vi "Set_Tunnel_Speed_server.vi"(3 "Tunnel Velocity m/s":dbl min=0.0 max=50.0 format="%.2f", 4 "Rig Name":string, 5 "Mode":T1, 6 "Client Name":string="G3_3 HD") -> (0 "Error String":string, 1 "Settling Time (s)":dbl format="%.2f", 2 "Valid Client":bool)   [LabVIEW 2013]
uses:
  ADAM Client/Sub VIs/ADAM Controls/Tunnel_speed_mode.ctl
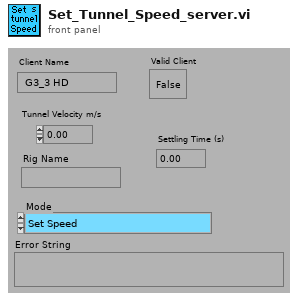
[diagram p1: front panel]
types:
  T1 = typedef "Tunnel_speed_mode.ctl" = enum16{"Set Speed", "Set Speed then wait", "Is tunnel speed allowable?"}
  T2 = typedef "Ch_description_ADAM.ctl" = cluster{"Ch Name":string, "Type":T3, "Function":T4, "Ch State":T5, "Calibration type":T6, "A":dbl, "B":dbl, "C":dbl, "D":dbl, "Comments":string, "Address":T7, "String":string, "Duty":u16}
  T3 = typedef "Module_type_ADAM.ctl" = string
  T4 = typedef "Function_ADAM.ctl" = enum16{"Analogue Input", "Digital Input", "Event counter", "Event rate", "Analogue Output", "Digital Output", "Relay Output"}
  T5 = typedef "Channel_State.ctl" = enum16{"On", "Off", "Always On", "Always Off"}
  T6 = typedef "Calib_type_ADAM.ctl" = enum16{"Raw", "Bx + A", "Cx^2 + Bx + A", "Dx^3 + Cx^2 + Bx + A", "In Band", "Hi-Tec Q", "Hi-Tec M_dot", "Text"}
  T7 = typedef "Address.ctl" = cluster{"Main":i32, "Ch.":i32, "Sub":i32, "Port Name":string}
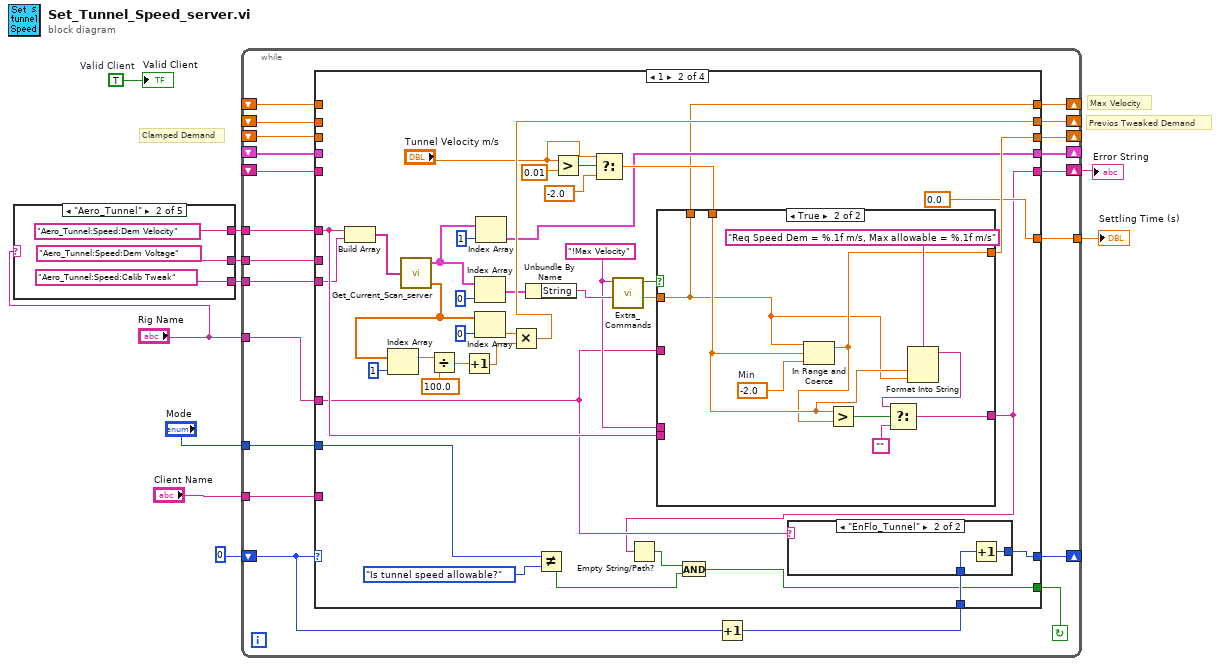
[diagram p0: block diagram]
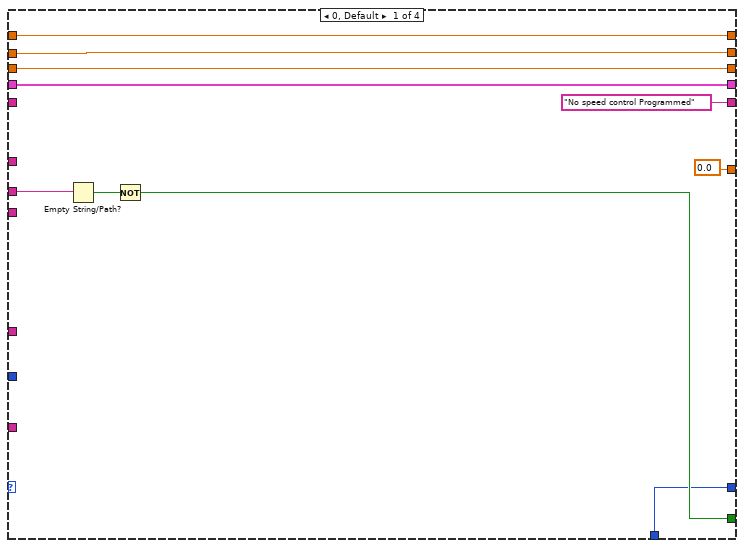
[diagram p2: hidden frame]
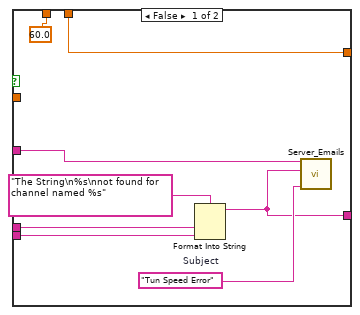
[diagram p4: hidden frame]
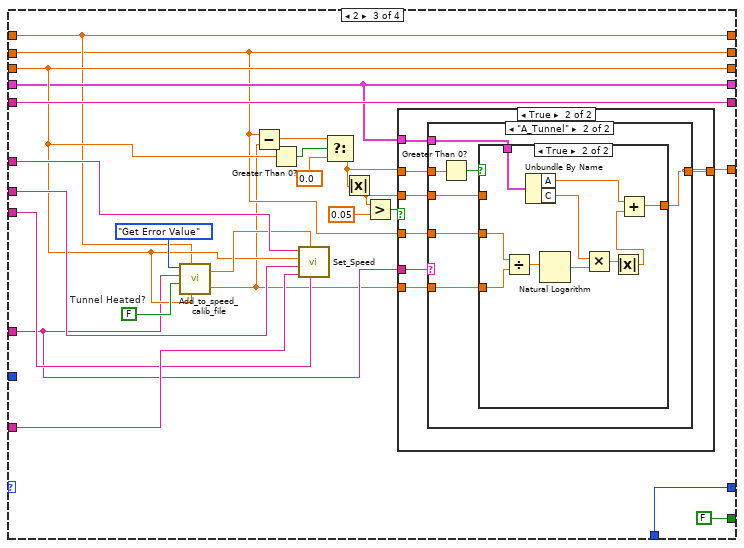
[diagram p5: hidden frame]
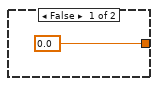
[diagram p6: hidden frame]
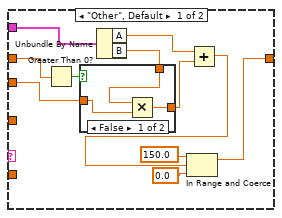
[diagram p7: hidden frame]
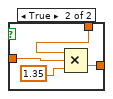
[diagram p8: hidden frame]
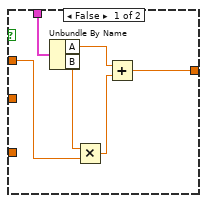
[diagram p9: hidden frame]
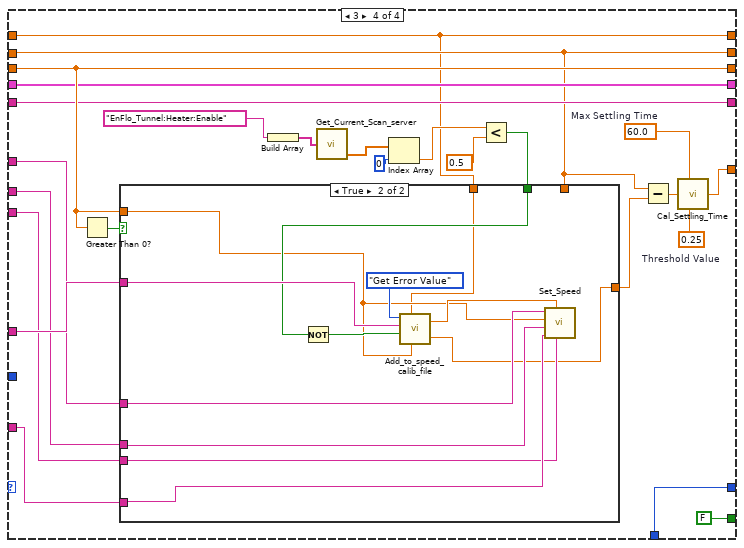
[diagram p10: hidden frame]
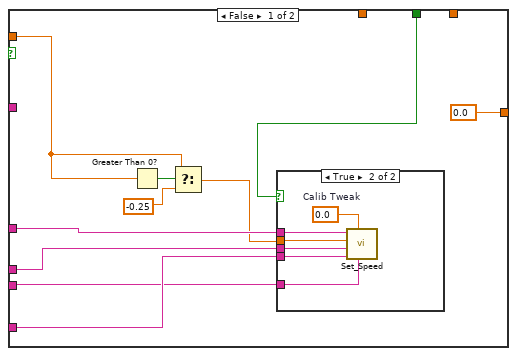
[diagram p11: hidden frame]
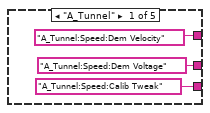
[diagram p13: hidden frame]
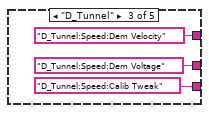
[diagram p14: hidden frame]
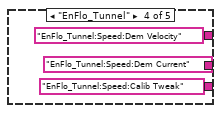
[diagram p15: hidden frame]
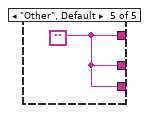
[diagram p16: hidden frame]
diagram:
  w10 = TRUE  # Valid Client
  # "Max Velocity"
  # "Previos Tweaked Demand"
  # "Clamped Demand"
  n1 = case shown="\"Aero_Tunnel\"" "Rig Name" {
    tunnel: ["A_Tunnel:Speed:Dem Velocity" "Aero_Tunnel:Speed:Dem Velocity" "D_Tunnel:Speed:Dem Velocity" "EnFlo_Tunnel:Speed:Dem Velocity" w23] -> w6
    tunnel: ["A_Tunnel:Speed:Dem Voltage" "Aero_Tunnel:Speed:Dem Voltage" "D_Tunnel:Speed:Dem Voltage" "EnFlo_Tunnel:Speed:Dem Current" w23] -> w3
    tunnel: ["A_Tunnel:Speed:Calib Tweak" "Aero_Tunnel:Speed:Calib Tweak" "D_Tunnel:Speed:Calib Tweak" "EnFlo_Tunnel:Speed:Calib Tweak" w23] -> w1
    frame "A_Tunnel" {
    }
    frame "Aero_Tunnel" {
    }
    frame "D_Tunnel" {
    }
    frame "EnFlo_Tunnel" {
    }
    frame "Other", Default {
      w23 = ""
    }
  }
  n2 = while {
    shift-left: _ -> [w26]
    shift-right: [w27] -> _
    tunnel: w1 -> [w28]
    shift-left: _ -> [w30]
    shift-right: [w29] -> _
    tunnel: [w31] -> w2
    tunnel: w3 -> [w33]
    shift-left: _ -> [w32]
    shift-right: [w36] -> w5
    shift-left: _ -> [w34]
    shift-right: [w37] -> _
    tunnel: w6 -> [w38]
    shift-left: 0 -> [w41]
    shift-right: [w40] -> _
    tunnel: "Client Name" -> [w43]
    tunnel: "Mode" -> [w44]
    tunnel: "Rig Name" -> [w42]
    shift-right: [w25] -> _
    shift-left: _ -> [w24]
    stop <- w35 continue-if-true
    n3 = Increment(x=w41) -> (x+1=w39:i32)
    n4 = case shown="1" w41 {
      tunnel: w34 -> [w50 _ w124 w199]
      tunnel: w44 -> [_ w83 _ _]
      tunnel: ["No speed control Programmed" w56 w131 w195] -> w36
      tunnel: w43 -> [_ _ w136 w209]
      tunnel: w42 -> [_ w75 w115 w208]
      tunnel: [w51 w78 w134 w200] -> w40
      tunnel: w39 -> [w51 w79 w134 w200]
      tunnel: w38 -> [_ w87 w133 w203]
      tunnel: [w50 w85 w124 w199] -> w37
      tunnel: [w52 w55 FALSE FALSE] -> w35
      tunnel: w33 -> [w54 _ w132 w202]
      tunnel: w32 -> [_ _ w131 w195]
      tunnel: [0.0 ("Settling Time") 0.0 ("Settling Time") w121 w197] -> w31
      tunnel: w30 -> [w48 _ w114 w190]
      tunnel: [w48 w66 w114 w190] -> w29
      tunnel: w28 -> [_ w74 w126 w193]
      tunnel: [w46 w60 w120 w191] -> w27
      tunnel: w26 -> [w46 _ w120 w191]
      tunnel: [w45 w59 w117 w187] -> w25
      tunnel: w24 -> [w45 _ w117 w187]
      frame 0, Default {
        n5 = Empty String/Path?(string/path=w54) -> (empty?=w53:bool)
        n6 = Not(x=w53) -> (.not. x?=w52:bool)
      }
      frame 1 {
        w88 = "!Max Velocity" ("Command")
        n7 = Build Array(w87, w74) -> (w92:string[])
        n8 = call "Get_Current_Scan_server.vi"("Desired Channels"=w92) -> ("Ch Description Array"=w61:T2[], "Numerical Values"=w72:dbl[])  [unwired: 1 out]
        n9 = Index Array(array=w72, index=1 ("Index")) -> (element=w71:dbl)
        n10 = Divide(x=w71, y=100.0) -> (x/y=w69:dbl)
        n11 = Increment(x=w69) -> (x+1=w67:dbl)
        n12 = Index Array(array=w61, index=0 ("Index")) -> (element=w63:T2)
        n13 = Index Array(array=w72, index=0 ("Index")) -> (element=w68:dbl)
        n14 = Index Array(array=w61, index=1 ("Index")) -> (element=w60:T2)
        n15 = Multiply(x=w68, y=w67) -> (x*y=w66:dbl)
        n16 = Unbundle By Name(w63) -> ("String"=w90:string)
        n17 = Not Equal?(x=w83, y=Tunnel_speed_mode."Is tunnel speed allowable?" ("Mode")) -> (x != y?=w57:bool)
        n18 = Greater?(x="Tunnel Velocity m/s", y=0.01) -> (0:w82:bool)
        n19 = Select(t="Tunnel Velocity m/s", s=w82, f=-2.0 ("t")) -> (s? t:f=w80:dbl)
        n20 = call "Extra_Commands.vi"("String to Search"=w90, "Command"=w88) -> ("Numeric Value"=w86:dbl, "Command Found"=w89:bool)  [unwired: 1 in, 3 out]
        n21 = case shown="True" w89 {
          tunnel: w75 -> [w97 _]
          tunnel: w88 -> [w102 _]
          tunnel: w87 -> [w101 _]
          tunnel: w86 -> [_ w104]
          tunnel: w80 -> [w99 w106]
          tunnel: [w99 w105] -> w85
          tunnel: [w98 w108] -> w56
          tunnel: [60.0 ("Numeric Value") w104] -> w59
          frame False {
            w103 = "Tun Speed Error"  # Subject
            n22 = Format Into String(format string="The String\n%s\nnot found for channel named %s" ("Format String"), w102, w101) -> (resulting string=w98:string)  [unwired: 2 in, 1 out]
            n23 = call "Server_Emails.vi"("Client Name Contains"=w97, "Message"=w98, "Subject"=w103) -> ()  [unwired: 2 in, 3 out]
          }
          frame True {
            w112 = -2.0  # Min
            n24 = In Range and Coerce(upper limit=w104, x=w106, lower limit=w112) -> (coerced(x)=w105:dbl)  [unwired: 1 out]
            n25 = Greater?(x=w106, y=w105) -> (0:w107:bool)
            n26 = Format Into String(format string="Req Speed Dem = %.1f m/s, Max allowable = %.1f m/s", w106, w104) -> (resulting string=w110:string)  [unwired: 2 in, 1 out]
            n27 = Select(t=w110, s=w107, f="") -> (s? t:f=w108:string)
          }
        }
        n28 = Empty String/Path?(string/path=w56) -> (empty?=w58:bool)
        n29 = And(x=w58, y=w57) -> (x .and. y?=w55:bool)
        n30 = case shown="\"EnFlo_Tunnel\"" w75 {
          tunnel: w79 -> [w93 w95]
          tunnel: [w93 w94] -> w78
          frame "Other", Default {
          }
          frame "EnFlo_Tunnel" {
            n31 = Increment(x=w95) -> (x+1=w94:i32)
          }
        }
      }
      frame 2 {
        w127 = FALSE  # Tunnel Heated?
        n32 = call "Add_to_speed_calib_file.vi"("Desired Velocity"=w124, "Max Velocity"=w117, "Tunnel Heated?"=w127, "Rig Name"=w115, "Mode"=enum16{"Add Row", "Get Error Value"}."Get Error Value") -> ("Tweaked Demand"=w113:dbl, "Calib Tweak %"=w125:dbl)  [unwired: 1 in]
        n33 = Subtract(x=w114, y=w113) -> (x-y=w129:dbl)
        n34 = Greater Than 0?(x=w124) -> (x > 0?=w116:bool)
        n35 = call "Set_Speed.vi"("Channel Name (Calib Tweak)"=w126, "Calib Tweak"=w125, "Client Name"=w136, "Channel Name (Volts/Amps)"=w132, "Demanded Velocity"=w124, "Channel Name (Velocity)"=w133) -> ()  [unwired: 1 in, 4 out]
        n36 = Select(t=w129, s=w116, f=0.0) -> (s? t:f=w119:dbl)
        n37 = Absolute Value(x=w119) -> (abs(x)=w118:dbl)
        n38 = Greater?(x=w118, y=0.05) -> (0:w122:bool)
        n39 = case shown="True" w122 {
          tunnel: w120 -> [_ w144]
          tunnel: [0.0 w141] -> w121
          tunnel: w119 -> [_ w143]
          tunnel: w118 -> [_ w142]
          tunnel: w115 -> [_ w140]
          tunnel: w114 -> [_ w139]
          tunnel: w113 -> [_ w138]
          frame False {
          }
          frame True {
            n40 = case shown="\"A_Tunnel\"" w140 {
              tunnel: w144 -> [w155 w166]
              tunnel: w143 -> [w150 w168]
              tunnel: w142 -> [w146 w167]
              tunnel: [w145 w165] -> w141
              tunnel: w139 -> [_ w164]
              tunnel: w138 -> [_ w163]
              frame "Other", Default {
                n41 = Greater Than 0?(x=w150) -> (x > 0?=w149:bool)
                n42 = Unbundle By Name(w155) -> ("A"=w154:dbl, "B"=w148:dbl)
                n43 = case shown="False" w149 {
                  tunnel: [w158 w159] -> w147
                  tunnel: w148 -> [w157 w162]
                  tunnel: w146 -> [w156 w161]
                  frame False {
                    n44 = Multiply(x=w157, y=w156) -> (x*y=w158:dbl)
                  }
                  frame True {
                    n45 = Compound Arithmetic op=MULTIPLY(w162, w161, 1.35 ("Min")) -> (w159:dbl)
                  }
                }
                n46 = Add(x=w154, y=w147) -> (x+y=w151:dbl)
                n47 = In Range and Coerce(upper limit=150.0 ("Max"), x=w151, lower limit=0.0 ("Min")) -> (coerced(x)=w145:dbl)  [unwired: 1 out]
              }
              frame "A_Tunnel" {
                n48 = Greater Than 0?(x=w168) -> (x > 0?=w169:bool)
                n49 = case shown="True" w169 {
                  tunnel: w167 -> [w171 _]
                  tunnel: w166 -> [w175 w185]
                  tunnel: [w170 w176] -> w165
                  tunnel: w164 -> [_ w183]
                  tunnel: w163 -> [_ w182]
                  frame False {
                    n50 = Unbundle By Name(w175) -> ("A"=w174:dbl, "B"=w172:dbl)
                    n51 = Multiply(x=w172, y=w171) -> (x*y=w173:dbl)
                    n52 = Add(x=w174, y=w173) -> (x+y=w170:dbl)
                  }
                  frame True {
                    n53 = Divide(x=w183, y=w182) -> (x/y=w184:dbl)
                    n54 = Unbundle By Name(w185) -> ("A"=w177:dbl, "C"=w180:dbl)
                    n55 = Natural Logarithm(1:w184) -> (0:w181:dbl)
                    n56 = Multiply(x=w180, y=w181) -> (x*y=w179:dbl)
                    n57 = Absolute Value(x=w179) -> (abs(x)=w178:dbl)
                    n58 = Add(x=w177, y=w178) -> (x+y=w176:dbl)
                  }
                }
              }
            }
          }
        }
      }
      frame 3 {
        w198 = 0.25  # Threshold Value
        w186 = 60.0  # Max Settling Time
        n59 = Greater Than 0?(x=w199) -> (x > 0?=w210:bool)
        n60 = Build Array("EnFlo_Tunnel:Heater:Enable") -> (w189:string[])
        n61 = call "Get_Current_Scan_server.vi"("Desired Channels"=w189) -> ("Numerical Values"=w188:dbl[])  [unwired: 2 out]
        n62 = Index Array(array=w188, index=0) -> (element=w204:dbl)
        n63 = Less?(x=w204, y=0.5) -> (x < y?=w194:bool)
        n64 = case shown="True" w210 {
          tunnel: w199 -> [w218 w228]
          tunnel: w203 -> [w217 w238]
          tunnel: w202 -> [w215 w237]
          tunnel: w209 -> [w214 w236]
          tunnel: w208 -> [_ w235]
          tunnel: w194 -> [w213 w233]
          tunnel: [0.0 w229] -> w192
          tunnel: w193 -> [w211 w231]
          tunnel: w190 -> [_ _]
          tunnel: w187 -> [_ w227]
          frame False {
            n65 = Greater Than 0?(x=w218) -> (x > 0?=w220:bool)
            n66 = Select(t=w218, s=w220, f=-0.25 ("t")) -> (s? t:f=w216:dbl)
            n67 = case shown="True" w213 {
              tunnel: w217 -> [_ w226]
              tunnel: w216 -> [_ w225]
              tunnel: w215 -> [_ w224]
              tunnel: w214 -> [_ w223]
              tunnel: w211 -> [_ w222]
              frame False {
              }
              frame True {
                w221 = 0.0  # Calib Tweak
                n68 = call "Set_Speed.vi"("Channel Name (Calib Tweak)"=w222, "Calib Tweak"=w221, "Client Name"=w223, "Channel Name (Volts/Amps)"=w224, "Demanded Velocity"=w225, "Channel Name (Velocity)"=w226) -> ()  [unwired: 1 in, 4 out]
              }
            }
          }
          frame True {
            n69 = Not(x=w233) -> (.not. x?=w232:bool)
            n70 = call "Add_to_speed_calib_file.vi"("Desired Velocity"=w228, "Max Velocity"=w227, "Tunnel Heated?"=w232, "Rig Name"=w235, "Mode"=enum16{"Add Row", "Get Error Value"}."Get Error Value") -> ("Tweaked Demand"=w229:dbl, "Calib Tweak %"=w230:dbl)  [unwired: 1 in]
            n71 = call "Set_Speed.vi"("Channel Name (Calib Tweak)"=w231, "Calib Tweak"=w230, "Client Name"=w236, "Channel Name (Volts/Amps)"=w237, "Demanded Velocity"=w228, "Channel Name (Velocity)"=w238) -> ()  [unwired: 1 in, 4 out]
          }
        }
        n72 = Subtract(x=w190, y=w192) -> (x-y=w196:dbl)
        n73 = call "Cal_Settling_Time.vi"("Max Settling Time"=w186, "Speed Tweak (m/s)"=w196, "Threshold Value"=w198) -> ("Required Settling Time"=w197:dbl)  [unwired: 2 out]
      }
    }
  }
  "Error String" <- w5
  "Settling Time (s)" <- w2
  "Valid Client" <- w10
